vi "Read SV.vi"(8 "error in (no error)":errorcluster, 11 "AEgIS Shared Variables in":refnum<class "Circus Shared Variables.lvclass">) -> (0 "error out":errorcluster, 2 "Variant":variant, 3 "AEgIS Shared Variables out":refnum<class "Circus Shared Variables.lvclass">)   [LabVIEW 2026, in "TALOS.lvlib" / "Classes.lvlib" / "Circus Shared Variables.lvclass"]
doc: "Use this VI to read a SV."
uses:
  Circus Shared Variables.lvclass
  Circus Shared Variables.lvclass/Circus Shared Variables.ctl
  Ancestor/Ancestor/Ancestor.lvclass/Ancestor.ctl
  Support VIs/Generate Error.vi
  FGV/Error Memory/Get Error Description.vi
  Support VIs/Get PC name.vi
  Ancestor/Ancestor/Read ID.vi
  Support VIs/Get Class Name.vi
  <vilib>/Utility/error.llb/Clear Errors.vi
  FGV/Error Memory/Error Memory Core.vi
  <vilib>/AdvancedString/Delimited String to 1D String Array.vi
  <vilib>/AdvancedString/Delimited String to 1D String Array (string).vi
  Support VIs/Circus Root Path.vi
  FGV/Error Memory/Error Crt Lvl checker.vi
  FGV/Error Memory/Error Memory Core.vi/40c8088d-b597-4017-91af-faa98e00292e.vi
  FGV/Error Memory/Error Memory Core.vi/d4a3ab98-063c-4e44-b43d-fbdcfe6c2be2.vi
  Support VIs/Global Memory.vi
  <vilib>/Utility/LVClass/Get LV Class Name.vi
  Support VIs/Is in Packed Library.vi
  Support VIs/TALOS Root path.vi
  Support VIs/Read CSV worksheet.vi
  Support VIs/Global Constants.vi
  <vilib>/Utility/error.llb/General Error Handler.vi
  Support VIs/Error Log.vi
  Ancestor/Ancestor/Ancestor.lvclass
  <vilib>/Comparison/Equal/Equal Functor/Equal Functor.lvclass
  TALOS.lvlib
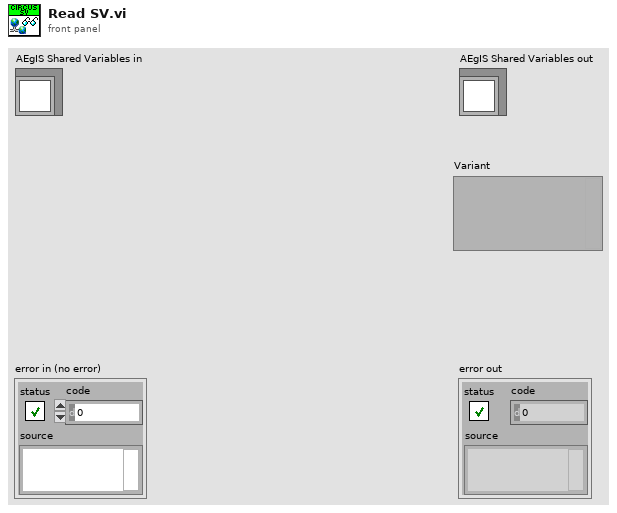
[diagram p1: front panel]
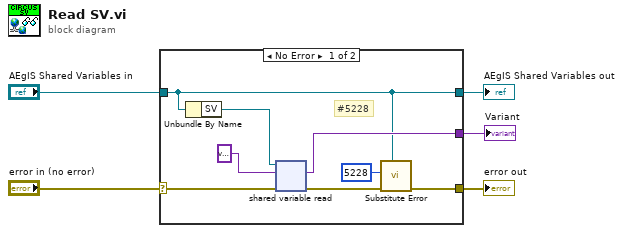
[diagram p0: block diagram]
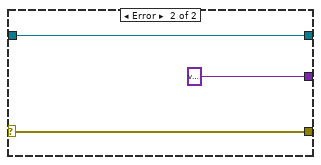
[diagram p2: hidden frame]
diagram:
  n1 = case shown="No Error" "error in (no error)" {
    selector: "error in (no error)" -> [w13 w16]
    tunnel: [w8 w16] -> w4
    tunnel: [w7 w15] -> w2
    tunnel: "AEgIS Shared Variables in" -> [w7 w15]
    tunnel: [w12 variant] -> w1
    frame No Error {
      # "#5228"
      n2 = Unbundle By Name(w7) -> ("SV"=w11:refnum<k21>)
      n3 = shared-variable-read(w11, w13, variant) -> (w9:errorcluster, w12:variant)  [unwired: 2 out]
      n4 = call "Substitute Error.vi"("LabVIEW Object"=w7, "error in (no error)"=w9, "Error Code"=5228) -> ("error out"=w8:errorcluster)  [unwired: 8 in]
    }
    frame Error {
    }
  }
  "error out" <- w4
  "AEgIS Shared Variables out" <- w2
  "Variant" <- w1
